vi "SerialCmd.vi"(6 "Show error dialog (T)":bool=TRUE, 9 "command":string="gcp\r", 10 "Return string skip chars (2)":i32=2, 11 "IMAQ Refnum in":refnum<k11>) -> (0 "Error":bool, 1 "String Read":string, 2 "CMD Success?":bool, 3 "IMAQ Session Out":refnum<k11>)   [LabVIEW 2011]
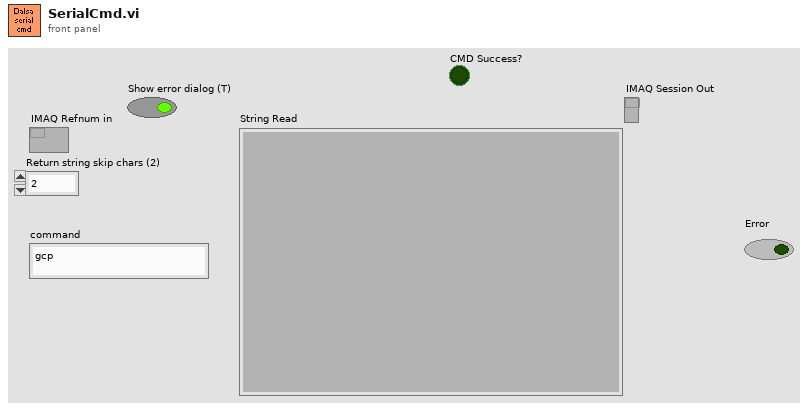
[diagram p1: front panel]
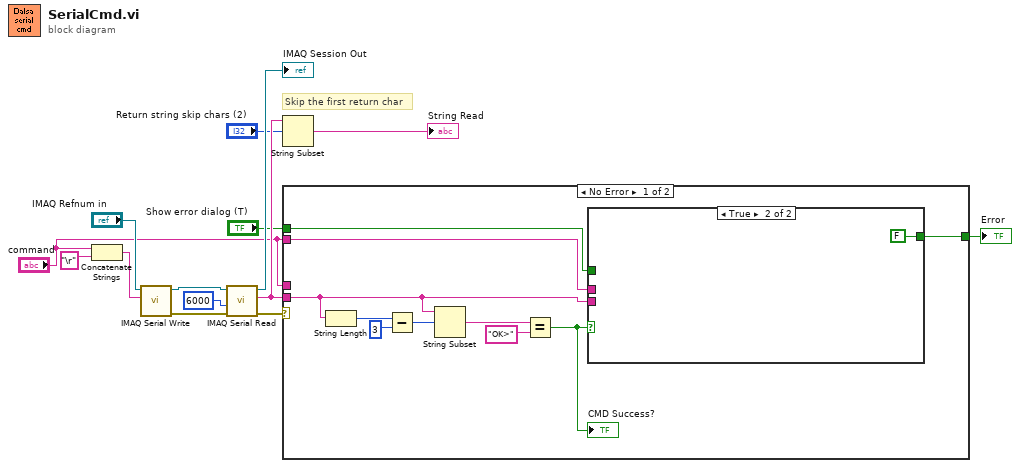
[diagram p0: block diagram]
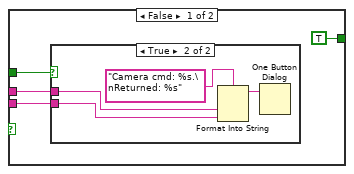
[diagram p2: hidden frame]
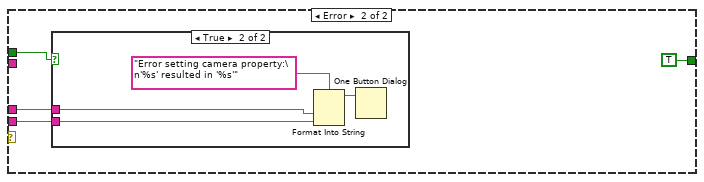
[diagram p4: hidden frame]
diagram:
  # "Skip the first return char"
  n1 = Concatenate Strings("command", "\r") -> (w4:string)
  n2 = call <vilib>:"IMAQ Serial Write.vi"("String to write"=w4, "IMAQ Session In"="IMAQ Refnum in") -> ("error out"=w13:errorcluster, "IMAQ Session Out"=w11:refnum<k11>)  [unwired: 2 in, 4 out]
  n3 = call <vilib>:"IMAQ Serial Read.vi"("error in (no error)"=w13, "Timeout"=u32 6000, "IMAQ Session In"=w11) -> ("error out"=w9:errorcluster, "String Read"=w8:string, "IMAQ Session Out"=→"IMAQ Session Out":refnum<k11>)  [unwired: 4 out]
  n4 = String Subset(string=w8, offset (0)="Return string skip chars (2)") -> (substring=→"String Read":string)  [unwired: 1 in]
  n5 = case shown="No Error" w9 {
    tunnel: w8 -> [w17 w36]
    tunnel: "command" -> [w18 _]
    tunnel: "command" -> [_ w37]
    tunnel: "Show error dialog (T)" -> [w15 w35]
    tunnel: [w16 TRUE ("Error")] -> w1
    frame No Error {
      n6 = String Length(string=w17) -> (length=w24:i32)
      n7 = Subtract(x=w24, y=3) -> (x-y=w22:i32)
      n8 = String Subset(string=w17, offset (0)=w22) -> (substring=w21:string)  [unwired: 1 in]
      n9 = Equal?(x=w21, y="OK>") -> (x = y?=w19:bool)
      "CMD Success?" <- w19
      n10 = case shown="True" w19 {
        tunnel: w18 -> [w28 _]
        tunnel: w17 -> [w27 _]
        tunnel: [TRUE ("Error") FALSE ("Error")] -> w16
        tunnel: w15 -> [w25 _]
        frame False {
          n11 = case shown="True" w25 {
            tunnel: w28 -> [_ w31]
            tunnel: w27 -> [_ w29]
            frame False {
            }
            frame True {
              n12 = Format Into String(format string="Camera cmd: %s.\nReturned: %s", w31, w29) -> (resulting string=w30:string)  [unwired: 2 in, 1 out]
              n13 = One Button Dialog(message=w30) -> ()  [unwired: 1 in, 1 out]
            }
          }
        }
        frame True {
        }
      }
    }
    frame Error {
      n14 = case shown="True" w35 {
        tunnel: w37 -> [_ w40]
        tunnel: w36 -> [_ w39]
        frame False {
        }
        frame True {
          n15 = Format Into String(format string="Error setting camera property:\n'%s' resulted in '%s'", w40, w39) -> (resulting string=w38:string)  [unwired: 2 in, 1 out]
          n16 = One Button Dialog(message=w38) -> ()  [unwired: 1 in, 1 out]
        }
      }
    }
  }
  "Error" <- w1
